vi "Find Object Item by Name.vi"(9 "Item Name":string, 10 "Offset":i32, 11 "JSON":string) -> (1 "JSON substring":string, 2 "Found":bool)   [LabVIEW 2013, in "JSON2.lvlib"]
uses:
  JSON2.lvlib
  Advance past colon.vi
  Advance past String.vi
  Advance past whitespace.vi
  Advance past comma.vi
  Advance past next JSON Value (COPY).vi
  Advance past Number.vi
  Advance past Array.vi
  Advance past Object.vi
  support/JSONtext support.lvlib
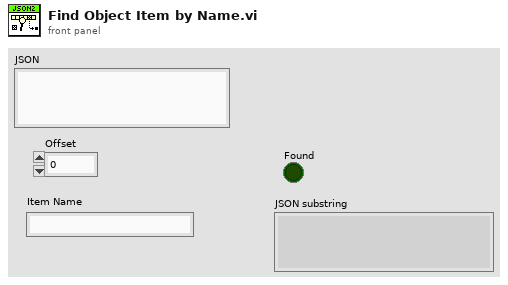
[diagram p1: front panel]
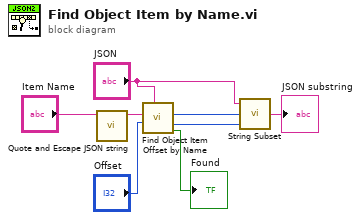
[diagram p0: block diagram]
diagram:
  n1 = call "Quote and Escape JSON string.vi"("Plain Text"="Item Name") -> ("<JSON>"=w4:string)  [unwired: 10 in]
  n2 = call "Find Object Item Offset by Name.vi"("JSON Object"="JSON", "Offset"="Offset", "Item Name <JSON>"=w4) -> ("Found"=→"Found":bool, "Offset past Item"=w1:i32, "Item start"=w6:i32)  [unwired: 5 in, 1 out]
  n3 = call "String Subset.vi"("Offset past match"=w1, "Value start in"=w6, "JSON"="JSON") -> ("substring"=→"JSON substring":string)  [unwired: 2 in]
